vi "LOG Message Loop.vi"(8 "error in (no error)":errorcluster) -> (0 "error out":errorcluster)   [LabVIEW 2020, in "LOG.lvlib"]
doc: "Message loop for handling messages pertaining to the acquisition of data from the hardware."
uses:
  LOG.lvlib
  support/PCT FGV CMD.ctl
  Acquisition State.ctl
  LOG Configuration.ctl
  support/Message Queue/Message Cluster.ctl
  support/Message Queue/Enqueue Message (Single).vi
  <vilib>/Utility/error.llb/Error Cluster From Error Code.vi
  <vilib>/ErrorRing/Error Ring.xnode
  support/Message Queue/Message Queue.lvlib
panel:
  out "# elements in queue":i32
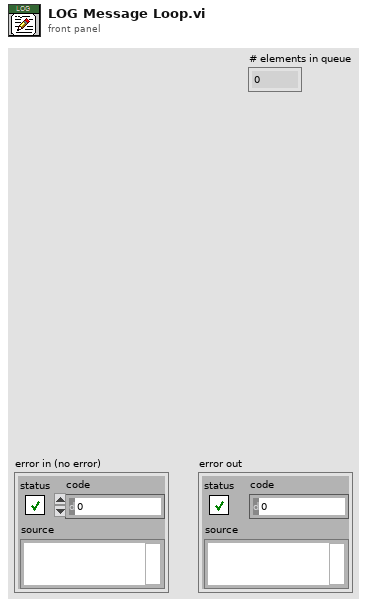
[diagram p1: front panel]
types:
  T1 = typedef "PCT FGV CMD.ctl" = enum16{"INIT", "GET", "SET"}
  T2 = typedef "Message Queue.lvlib/All Message Queues.ctl" = cluster{"UI":refnum<queue>, "Logging":refnum<queue>, "LOG":refnum<queue>, "ALARM":refnum<queue>, "Test":refnum<queue>, "Answer":refnum<queue>, "PLC":refnum<queue>, "DB":refnum<queue>, "Report":refnum<queue>, "OPC":refnum<queue>, "Procedure":refnum<queue>, "PalmSens":refnum<queue>, "SYS 7000 Reader":refnum<queue>, "SWITCH":refnum<queue>, "MOTOR":refnum<queue>, "MOTION":refnum<queue>, "HIDEN":refnum<queue>, "VALVE":refnum<queue>, "MFC":refnum<queue>, "PUMP IN":refnum<queue>, "PUMP OUT":refnum<queue>}
  T3 = typedef "LOG.lvlib/LOG Configuration.ctl" = cluster{"LOG REF":refnum<vi>, "Writer Queue":refnum<queue>, "Log Path":path, "LOG":bool}
  T4 = typedef "LOG.lvlib/Acquisition State.ctl" = enum16{"Idle", "Initialized"}
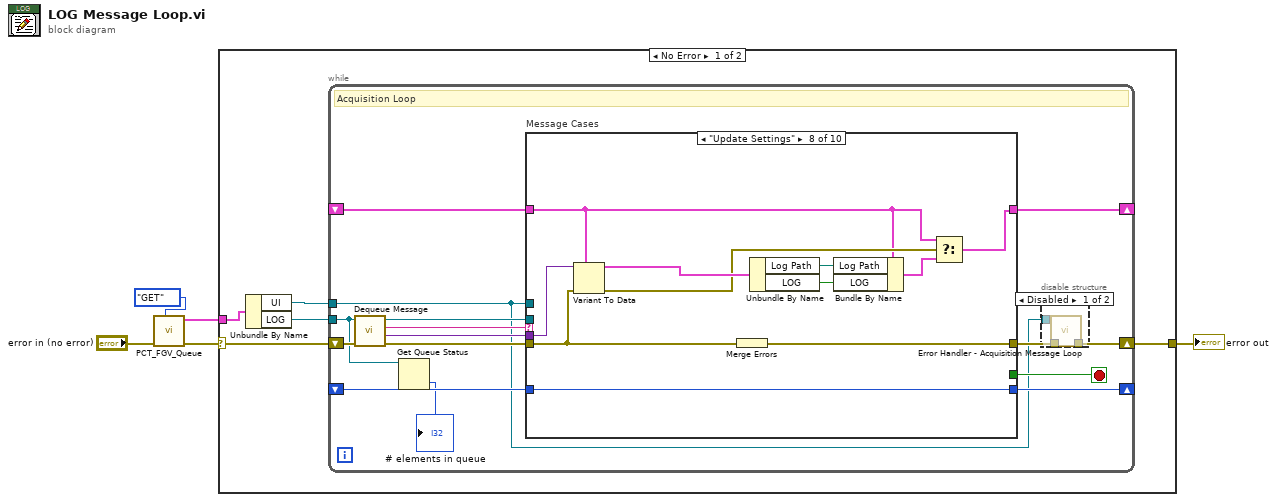
[diagram p0: block diagram]
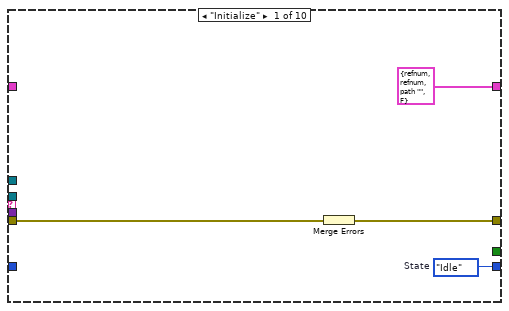
[diagram p3: hidden frame]
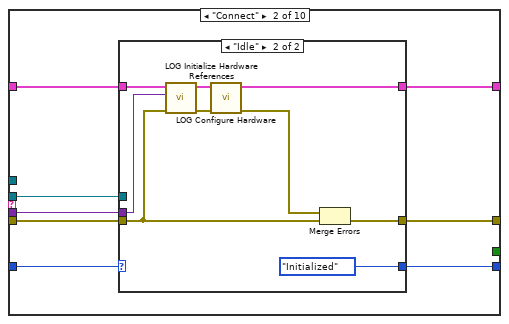
[diagram p4: hidden frame]
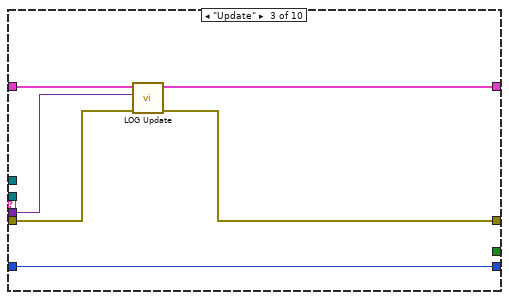
[diagram p6: hidden frame]
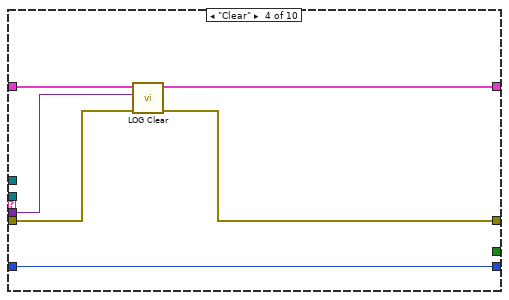
[diagram p7: hidden frame]
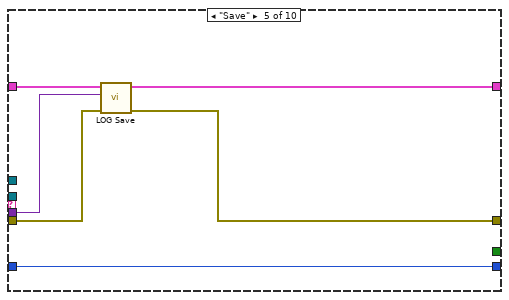
[diagram p8: hidden frame]
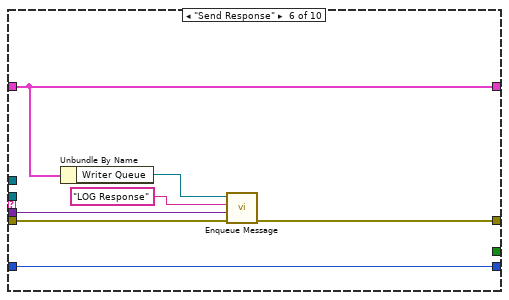
[diagram p9: hidden frame]
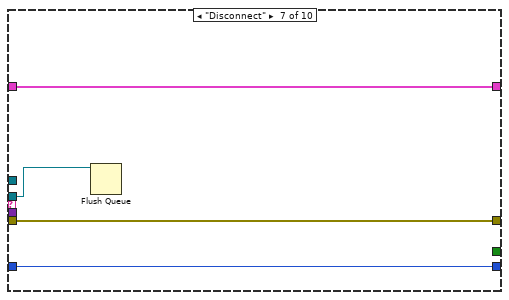
[diagram p10: hidden frame]
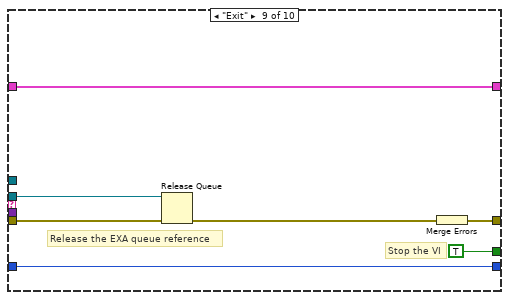
[diagram p11: hidden frame]
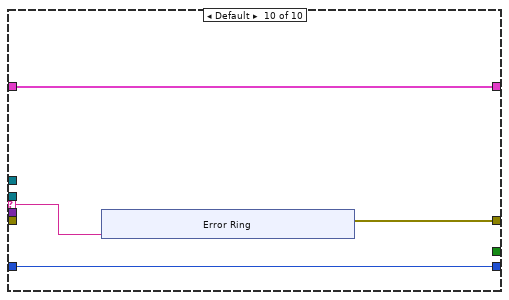
[diagram p12: hidden frame]
diagram:
  n1 = call "PCT_FGV_Queue.vi"("CMD"=PCT_FGV_CMD."GET", "error in (no error)"="error in (no error)") -> ("error out"=w2:errorcluster, "Message Queues out"=w1:T2)  [unwired: 8 in]
  n2 = case shown="No Error" w2 {
    selector: w2 -> [w7 w111]
    tunnel: w1 -> [w10 _]
    tunnel: [w8 w111] -> w5
    frame No Error {
      n3 = Unbundle By Name(w10) -> ("UI"=w6:refnum<queue>, "LOG"=w9:refnum<queue>)
      n4 = while {
        tunnel: w9 -> [w12]
        shift-right: [w24] -> _
        shift-left: _ -> [w25]
        shift-right: [w16] -> w8
        shift-left: w7 -> [w22]
        tunnel: w6 -> [w13]
        shift-right: [w17] -> _
        shift-left: _ -> [w18]
        stop <- w23 stop-if-true
        # "Acquisition Loop"
        n5 = call "Dequeue Message.vi"("error in (no error)"=w22, "Message Queue"=w12) -> ("error out"=w21:errorcluster, "Message Data"=w19:variant, "Message"=w20:string, "dup Message Queue"=w14:refnum<queue>)  [unwired: 6 in]
        n6 = Get Queue Status(queue=w12) -> (# elements in queue=→"# elements in queue":i32)  [unwired: 2 in, 7 out]
        n7 = case "Message Cases" shown="\"Update Settings\"" w20 {
          selector: w20 -> [_ _ _ _ _ _ _ _ _ w100]
          tunnel: w14 -> [_ w37 _ _ _ _ w78 _ w94 _]
          tunnel: w21 -> [w31 w38 w54 w60 w66 w75 w80 w89 w96 _]
          tunnel: [w32 w40 w53 w59 w65 w74 w80 w92 w98 w101] -> w15
          tunnel: w25 -> [_ w39 w55 w61 w67 w72 w79 w83 w97 w103]
          tunnel: [T3 {"LOG REF"=refnum, "Writer Queue"=refnum, "Log Path"=path "", "LOG"=FALSE} ("Data Cluster") w36 w56 w62 w68 w72 w79 w90 w97 w103] -> w24
          tunnel: [_ _ _ _ _ _ _ _ TRUE _] -> w23
          tunnel: w19 -> [_ w33 w57 w63 w69 w73 _ w91 _ _]
          tunnel: w13 -> [_ _ _ _ _ _ _ _ _ _]
          tunnel: w18 -> [_ w34 w58 w64 w70 w76 w81 w88 w93 w102]
          tunnel: [w30 w35 w58 w64 w70 w76 w81 w88 w93 w102] -> w17
          frame "Initialize" {
            w30 = Acquisition_State."Idle"  # State
            # "Initialize  - Initialize is currently a no-op.  The hardware initialization takes place in the 'Start' message."
            n8 = Merge Errors(w31) -> (w32:errorcluster)
          }
          frame "Connect" {
            # "Start - Configure and start the acquisition."
            n9 = case shown="\"Idle\"" w34 {
              selector: w34 -> [w41 _]
              tunnel: [w42 w52] -> w40
              tunnel: w39 -> [w43 w51]
              tunnel: w38 -> [w42 w45]
              tunnel: w37 -> [_ _]
              tunnel: [w43 w47] -> w36
              tunnel: [w41 Acquisition_State."Initialized" ("Acquisition State")] -> w35
              tunnel: w33 -> [_ w44]
              frame "Initialized" {
                # "The system is already acquiring. Ignore the \"Start\" message."
              }
              frame "Idle" {
                # "If the system is idle, start the acquisition."
                n10 = call "LOG Initialize Hardware References.vi"("error in (no error)"=w45, "Message Data"=w44, "Hardware Resources in"=w51) -> ("error out"=w50:errorcluster, "Hardware Resources out"=w48:T3)  [unwired: 7 in]
                n11 = call "LOG Configure Hardware.vi"("error in (no error)"=w50, "Hardware Resources in"=w48) -> ("error out"=w49:errorcluster, "Hardware Resources out"=w47:T3)  [unwired: 8 in]
                n12 = Merge Errors(w49, w45) -> (w52:errorcluster)
              }
            }
          }
          frame "Update" {
            # "Start - Configure and start the acquisition."
            n13 = call "LOG Update.vi"("error in (no error)"=w54, "Message Data"=w57, "Data Cluster"=w55) -> ("error out"=w53:errorcluster, "Data Cluster out"=w56:T3)  [unwired: 7 in]
          }
          frame "Clear" {
            # "Start - Configure and start the acquisition."
            n14 = call "LOG Clear.vi"("error in (no error)"=w60, "Message Data"=w63, "Data Cluster"=w61) -> ("error out"=w59:errorcluster, "Data Cluster out"=w62:T3)  [unwired: 7 in]
          }
          frame "Save" {
            # "Start - Configure and start the acquisition."
            n15 = call "LOG Save.vi"("error in (no error)"=w66, "Message Data"=w69, "Data Cluster"=w67) -> ("error out"=w65:errorcluster, "Data Cluster out"=w68:T3)  [unwired: 7 in]
          }
          frame "Send Response" {
            # "Acquire - Acquire data from the hardware. Since this is a continuous acquisition, this message will always message itself to run again."
            n16 = Unbundle By Name(w72) -> ("Writer Queue"=w71:refnum<queue>)
            n17 = call-poly "Enqueue Message.vi"("error in (no error)"=w75, "Message Data"=w73, "Message"="LOG Response", "Message Queue"=w71) -> ("error out"=w74:errorcluster)  [unwired: 6 in, 1 out]
          }
          frame "Disconnect" {
            # "Acquire - Acquire data from the hardware. Since this is a continuous acquisition, this message will always message itself to run again."
            n18 = Flush Queue(queue=w78) -> ()  [unwired: 1 in, 3 out]
          }
          frame "Update Settings" {
            # "New settings are available, update the current ones stored in the shift register with the settings sent as part of the message"
            n19 = Variant To Data(error in=w89, type=w83, Variant=w91) -> (data=w87:T3, error out=w84:errorcluster)
            n20 = Merge Errors(w89) -> (w92:errorcluster)
            n21 = Unbundle By Name(w87) -> ("Log Path"=w86:path, "LOG"=w82:bool)
            n22 = Bundle By Name(cluster=w83, "Log Path"=w86, "LOG"=w82) -> (w85:T3)
            n23 = Select(t=w83, s=w84, f=w85) -> (s? t:f=w90:T3)
          }
          frame "Exit" {
            # "Release the EXA queue reference"
            # "Stop the VI"
            # "Exit - Send the Exit message to the UI Message Handler."
            n24 = Release Queue(queue=w94, error in (no error)=w96) -> (error out=w95:errorcluster)  [unwired: 1 in, 2 out]
            n25 = Merge Errors(w95) -> (w98:errorcluster)
          }
          frame Default {
            # "'Default' case only runs if there is a message that isn't defined in any of the other cases.  Output a programming error."
            n26 = xnode "Error Ring"("parameter 0"=w100) -> ("error out"=w101:errorcluster)
          }
        }
        n27 = disable-structure shown="Disabled" {
          disable-tunnel: [w28 _] -> w16
          disable-tunnel: w15 -> [w27 _]
          disable-tunnel: w13 -> [w26 _]
          frame Disabled {
            n28 = call "Error Handler - Acquisition Message Loop.vi"("error in (no error)"=w27, "Message Queue"=w26) -> ("dup error in"=w28:errorcluster)  [unwired: 8 in, 1 out]
          }
          frame Enabled {
          }
        }
      }
    }
    frame Error {
    }
  }
  "error out" <- w5
